vi "FGV_Counter.vi"(9 "increment":bool) -> (1 "counter":T1)   [LabVIEW 2021]
uses:
  Counter.ctl
panel:
  out "Numeric":dbl
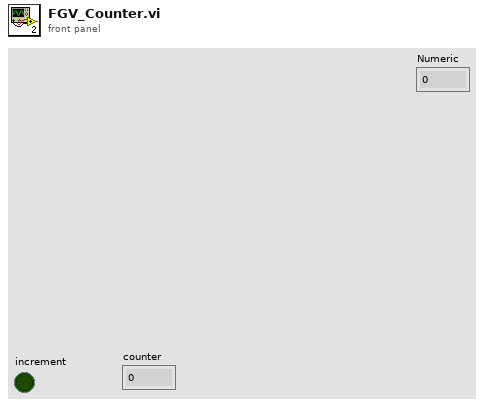
[diagram p1: front panel]
types:
  T1 = typedef "Counter.ctl" = u8
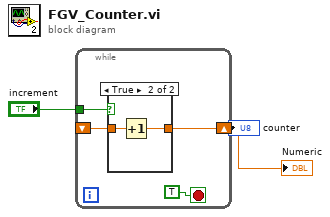
[diagram p0: block diagram]
diagram:
  n1 = while {
    shift-right: [w4] -> w1
    shift-left: _ -> [w5]
    tunnel: "increment" -> [w3]
    stop <- TRUE stop-if-true
    n2 = case shown="True" w3 {
      tunnel: w5 -> [w7 w9]
      tunnel: [w7 w8] -> w4
      frame False {
      }
      frame True {
        n3 = Increment(x=w9) -> (x+1=w8:dbl)
      }
    }
  }
  "counter" <- w1
  "Numeric" <- w1
